vi "test_abort.vi"   [LabVIEW 2020]
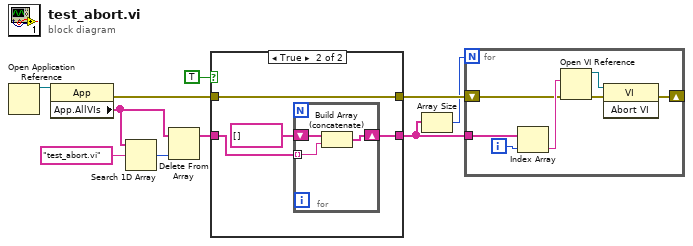
[diagram p0: block diagram]
diagram:
  n1 = Open Application Reference() -> (3:w3:refnum<vi>)  [unwired: 4 in, 1 out]
  n2 = property class="App"(reference=w3) -> (error out=w7:errorcluster, "App.AllVIs"=w4:string[])  [unwired: 1 in, 1 out]
  n3 = Search 1D Array(1D array=w4, element="test_abort.vi") -> (index of element=w5:i32)  [unwired: 1 in]
  n4 = Delete From Array(array=w4, index=w5) -> (array with subset deleted=w6:string[])  [unwired: 1 in, 1 out]
  n5 = case shown="True" TRUE {
    tunnel: w6 -> [w11 w16]
    tunnel: w7 -> [w12 w13]
    tunnel: [w11 w14] -> w9
    tunnel: [w12 w13] -> w10
    frame False {
    }
    frame True {
      n6 = for {
        tunnel: w16 -> [w18] mode=indexing
        shift-right: [w17] -> w14
        shift-left: string[] [] -> [w19]
        n7 = Build Array (concatenate)(w19, w18) -> (w17:string[])
      }
    }
  }
  n8 = Array Size(array=w9) -> (size(s)=w8:i32)
  n9 = for {
    N: w8 -> [_]
    tunnel: w9 -> [w25]
    shift-right: [w20] -> _
    shift-left: w10 -> [w21]
    i -> [w26]
    n10 = Index Array(array=w25, index=w26) -> (element=w24:string)
    n11 = Open VI Reference(vi path=w24, error in (no error)=w21) -> (vi reference=w23:refnum<vi>, error out=w22:errorcluster)  [unwired: 4 in]
    n12 = invoke class="VI" method="Abort VI"(reference=w23, error in=w22) -> (error out=w20:errorcluster)  [unwired: 1 in, 2 out]
  }
